vi "PipeLine Gaussian Filter(3x3).vi"(4 "Pixel Data":u8, 5 "X":i16, 6 "Height":u32, 7 "Line2":refnum<k21>, 8 "Y":i16, 9 "DV":bool, 10 "Line3":refnum<k21>, 11 "Line1":refnum<k21>) -> (2 "Output Pixel":fxp<+,12,12>)   [LabVIEW 2016]
uses:
  <vilib>/rvi/DataTransferAndStorage/Container/Common/niFpgaContainerExecOnDevCompGetState.vi
  <vilib>/rvi/Emulation/niFpgaEmulationIsFPGAContextNoSignature.vi
  <vilib>/rvi/DataTransferAndStorage/Container/Common/niFpgaContainerGetUniqueNameForEmu.vi
  <vilib>/rvi/Emulation/niFpgaProcessEmulError.vi
  <vilib>/rvi/Emulation/niFpgaSctlEmulationGetInTimedLoop.vi
  <vilib>/rvi/errors/nirviReportUnexpectedCaseInternalError (U32).vi
  <vilib>/rvi/Memory/Memory_Emulation/niFpgaMemoryEmulationCacheClearOnFirstRun.vi
  <vilib>/rvi/Memory/Memory_Emulation/nirvimemoryEmulationManagerCache_MakeExclusive.vi
  <vilib>/rvi/Memory/Memory_Emulation/niFpgaMemoryEmulationValidateCache.vi
  <vilib>/rvi/Memory/Memory_Emulation/nirvimemoryEmulationManagerCache_InsertValue.vi
  <vilib>/Utility/error.llb/Clear Errors.vi
  <vilib>/rvi/Memory/Memory_Emulation/nirvimemoryEmulationManagerCache_ReleaseExclusive.vi
  <vilib>/rvi/Memory/Memory_Emulation/nirvimemoryEmulationManagerCache_GetValue.vi
  <vilib>/rvi/Memory/Memory_Emulation/nirvimemoryEmulationManagerCache_SetValue.vi
  <vilib>/rvi/Emulation/niFpgaSctlEmulationResourceMgr.vi
  <vilib>/rvi/DataTransferAndStorage/Container/Common/niFpgaContainerSetEmuInfo.vi
  <vilib>/rvi/eio/common/nirviEmuReportErrorAndStop.vi
  <vilib>/rvi/DataTransferAndStorage/Container/XNode/niFpgaContainer.xnode
  <vilib>/rvi/Memory/Memory_Emulation/niFpgaMemoryEmulationRefIn.vi
  <vilib>/rvi/LocalResourceManager/LocalResourceManager.xnode
  <vilib>/rvi/DataTransferAndStorage/Register/Emulation/niFpgaRegisterEmulationRefIn.vi
panel:
  out "Memory Out":refnum<k21>
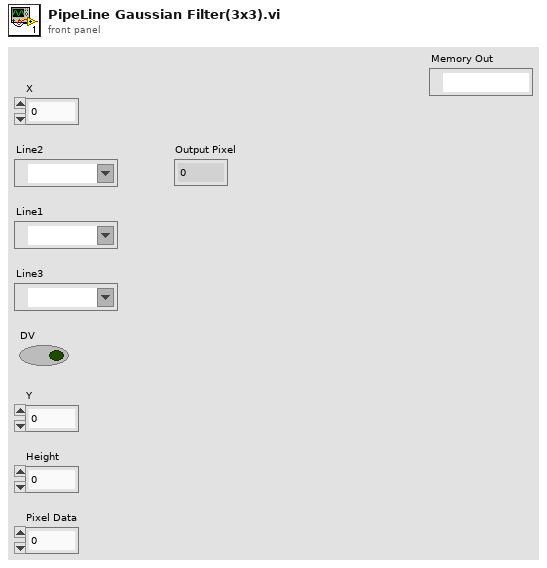
[diagram p1: front panel]
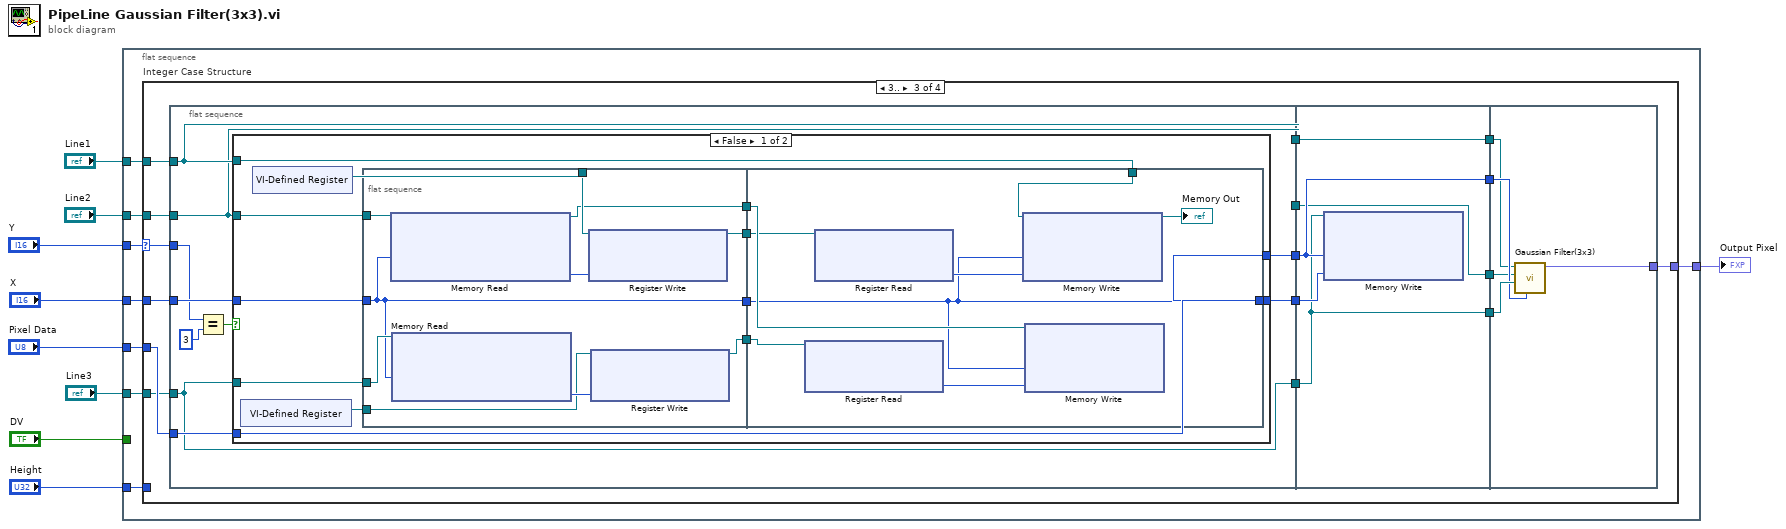
[diagram p0: block diagram]
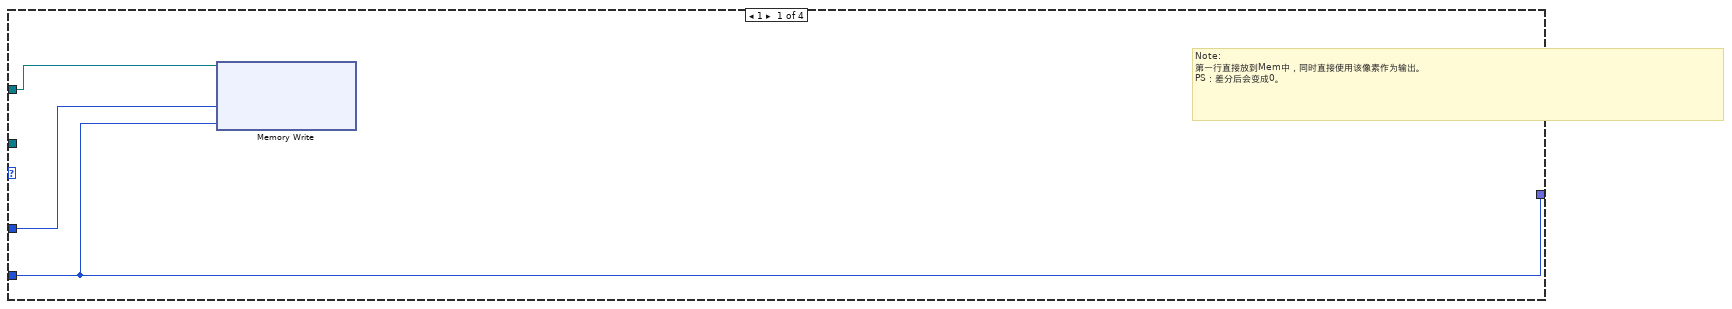
[diagram p2: hidden frame]
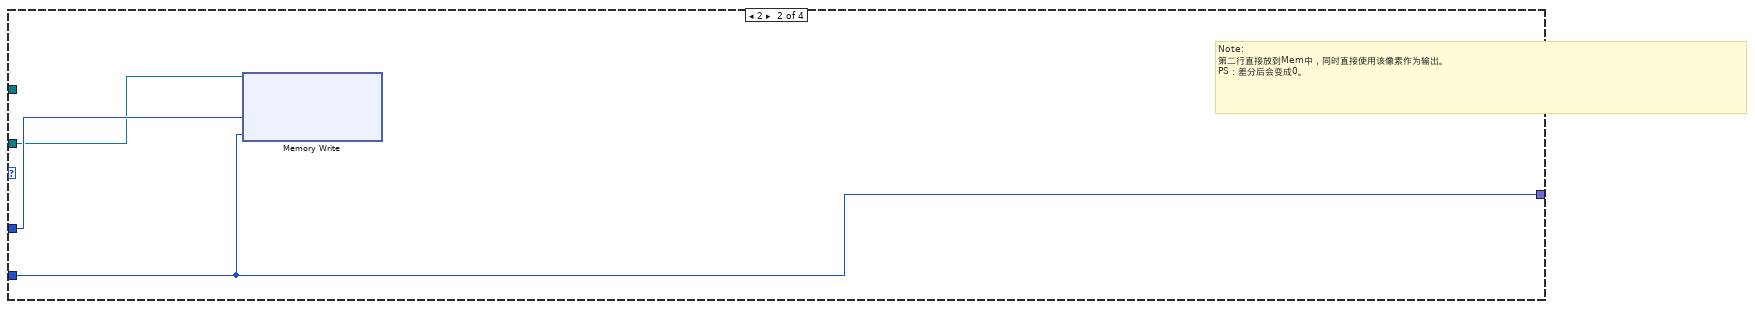
[diagram p3: hidden frame]
diagram:
  n1 = flat-sequence {
    tunnel: "Y" -> [w17]
    tunnel: "X" -> [w16]
    tunnel: "Pixel Data" -> [w15]
    tunnel: [w14] -> w6
    tunnel: "Height" -> [w13]
    tunnel: "Line1" -> [w12]
    tunnel: "Line2" -> [w11]
    tunnel: "Line3" -> [w10]
    tunnel: "DV" -> [_]
    frame #0 {
      n2 = case "Integer Case Structure" shown="3.." w17 {
        selector: w17 -> [_ _ w31 _]
        tunnel: w16 -> [w20 w23 w39 _]
        tunnel: w15 -> [w19 w22 w38 w92]
        tunnel: [w19 w22 w35 w92] -> w14
        tunnel: w13 -> [_ _ _ _]
        tunnel: w12 -> [w18 _ w28 _]
        tunnel: w11 -> [_ w21 w27 _]
        tunnel: w10 -> [_ _ w26 _]
        frame 1 {
          # "Note: \n第一行直接放到Mem中，同时直接使用该像素作为输出。\nPS：差分后会变成0。"
          # "This diagram executes if the integer value is 0, 2, or any number between 4 and 9 (inclusive)."
          n3 = xnode "Memory Write"("Memory In"=w18, "Address"=w20, "Data"=w19) -> ()  [unwired: 1 out]
        }
        frame 2 {
          # "Note: \n第二行直接放到Mem中，同时直接使用该像素作为输出。\nPS：差分后会变成0。"
          n4 = xnode "Memory Write"("Address"=w23, "Data"=w22, "Memory In"=w21) -> ()  [unwired: 1 out]
        }
        frame 3.. {
          n5 = flat-sequence {
            tunnel: w38 -> [w48]
            tunnel: w39 -> [w49]
            tunnel: w26 -> [w44]
            tunnel: [w44] -> w34
            tunnel: [w46] -> w33
            tunnel: [w47] -> w32
            tunnel: w31 -> [w41]
            tunnel: w28 -> [w45]
            tunnel: [w45] -> w29
            tunnel: w27 -> [w43]
            tunnel: [w43] -> w24
            tunnel: [w85] -> w37
            tunnel: [w84] -> w36
            tunnel: w34 -> [w84]
            tunnel: w33 -> [w85]
            tunnel: w32 -> [w86]
            tunnel: [w83] -> w30
            tunnel: w29 -> [w83]
            tunnel: [w82] -> w25
            tunnel: w24 -> [w82]
            tunnel: w37 -> [w90]
            tunnel: w36 -> [w91]
            tunnel: [w89] -> w35
            tunnel: w30 -> [w88]
            tunnel: w25 -> [w87]
            frame #0 {
              n6 = Equal?(x=w41, y=i16 3) -> (x = y?=w42:bool)
              n7 = case shown="False" w42 {
                tunnel: w49 -> [w59 w80]
                tunnel: w48 -> [w55 w81]
                tunnel: [w55 w81] -> w47
                tunnel: [w54 w80] -> w46
                tunnel: w45 -> [w56 _]
                tunnel: w44 -> [w61 _]
                tunnel: w43 -> [w60 _]
                frame False {
                  n8 = xnode "VI-Defined Register"() -> ("Register Out"=w58:refnum<k21>)
                  n9 = xnode "VI-Defined Register"() -> ("Register Out"=w57:refnum<k21>)
                  n10 = flat-sequence {
                    tunnel: w61 -> [w71]
                    tunnel: w60 -> [w65]
                    tunnel: w59 -> [w67]
                    tunnel: w57 -> [w70]
                    tunnel: w58 -> [w66]
                    tunnel: [w67] -> w53
                    tunnel: [w64] -> w52
                    tunnel: [w63] -> w51
                    tunnel: [w62] -> w50
                    tunnel: w56 -> [w72]
                    tunnel: [w77] -> w54
                    tunnel: w50 -> [w74]
                    tunnel: w51 -> [w76]
                    tunnel: w52 -> [w78]
                    tunnel: w53 -> [w77]
                    frame #0 {
                      n11 = xnode "Memory Read"("Address"=w67, "Memory In"=w65) -> ("Data"=w69:u8, "Memory Out"=w64:refnum<k21>)
                      n12 = xnode "Memory Read"("Address"=w67, "Memory In"=w71) -> ("Data"=w68:u8)  [unwired: 1 out]
                      n13 = xnode "Register Write"("Data"=w69, "Register In"=w70) -> ("Register Out"=w62:refnum<k21>)
                      n14 = xnode "Register Write"("Data"=w68, "Register In"=w66) -> ("Register Out"=w63:refnum<k21>)
                    }
                    frame #1 {
                      n15 = xnode "Register Read"("Register In"=w76) -> ("Data"=w75:i16)  [unwired: 1 out]
                      n16 = xnode "Register Read"("Register In"=w74) -> ("Data"=w79:i16)  [unwired: 1 out]
                      n17 = xnode "Memory Write"("Memory In"=w72, "Address"=w77, "Data"=w79) -> ("Memory Out"=→"Memory Out":refnum<k21>)
                      n18 = xnode "Memory Write"("Address"=w77, "Data"=w75, "Memory In"=w78) -> ()  [unwired: 1 out]
                    }
                  }
                }
                frame True {
                }
              }
            }
            frame #1 {
              n19 = xnode "Memory Write"("Address"=w85, "Data"=w86, "Memory In"=w84) -> ()  [unwired: 1 out]
            }
            frame #2 {
              n20 = call "Gaussian Filter(3x3).vi"("Input ColNum"=w90, "Line 3"=w91, "Line 2"=w87, "Line 1"=w88) -> ("Output"=w89:fxp<+,12,12>)  [unwired: 7 in]
            }
          }
        }
        frame Default {
          # "This diagram executes if the integer value is anything other than what is specified in the other cases of this case structure."
        }
      }
    }
  }
  "Output Pixel" <- w6
